vi "HEWH GEA3.vi"(8 "error in":errorcluster, 11 "Message Queues out":T4) -> (0 "error out":errorcluster)   [LabVIEW 2023]
uses:
  Tenney/support/Message Queue/All Message Queues.ctl
  Tenney/support/Message Queue/Message Cluster.ctl
  Type Definitions/HEWH GEA3 Data.ctl
  Drivers/GEA3 Toolkit/LabVIEW GEA3 Rev2 API Toolkit LV2016/Water Heating Specific/Type Definitions/GEA3 HEWH ERD Data.ctl
  Drivers/GEA3 Toolkit/LabVIEW GEA3 Rev2 API Toolkit LV2016/Water Heating Specific/Type Definitions/GEA3 HEWH Mixing Valve.ctl
  Type Definitions/HEWH GEA3 Board ID.ctl
  Drivers/GEA3 Toolkit/LabVIEW GEA3 Rev2 API Toolkit LV2016/type defs/ERD Write Data In.ctl
  Drivers/GEA3 Toolkit/LabVIEW GEA3 Rev2 API Toolkit LV2016/type defs/Data Type.ctl
  Utility/Save File/File Setup (Public)/Type Definition/Save File HEWH Heating Control Mode.ctl
  Drivers/GEA3 Toolkit/LabVIEW GEA3 Rev2 API Toolkit LV2016/Water Heating Specific/Type Definitions/GEA3 HEWH Personality.ctl
  FVIR and LDO/support/Message Queue/Enqueue Message (Single).vi
  FVIR and LDO/support/Message Queue/Message Queue.lvlib
  Drivers/GEA3 Toolkit/LabVIEW GEA3 Rev2 API Toolkit LV2016/library/GEA2_Toolkit.lvlib
  Utility/Save File/File Setup.lvlib
  Tenney/support/Message Queue/Tenney Message Queue.lvlib
panel:
  out "Loop Count":i32
  out "GEA3 Data":T1
  out "Pink Bean Board ID":string
  in  "Debug":bool
  out "Debug":string[](array[string])
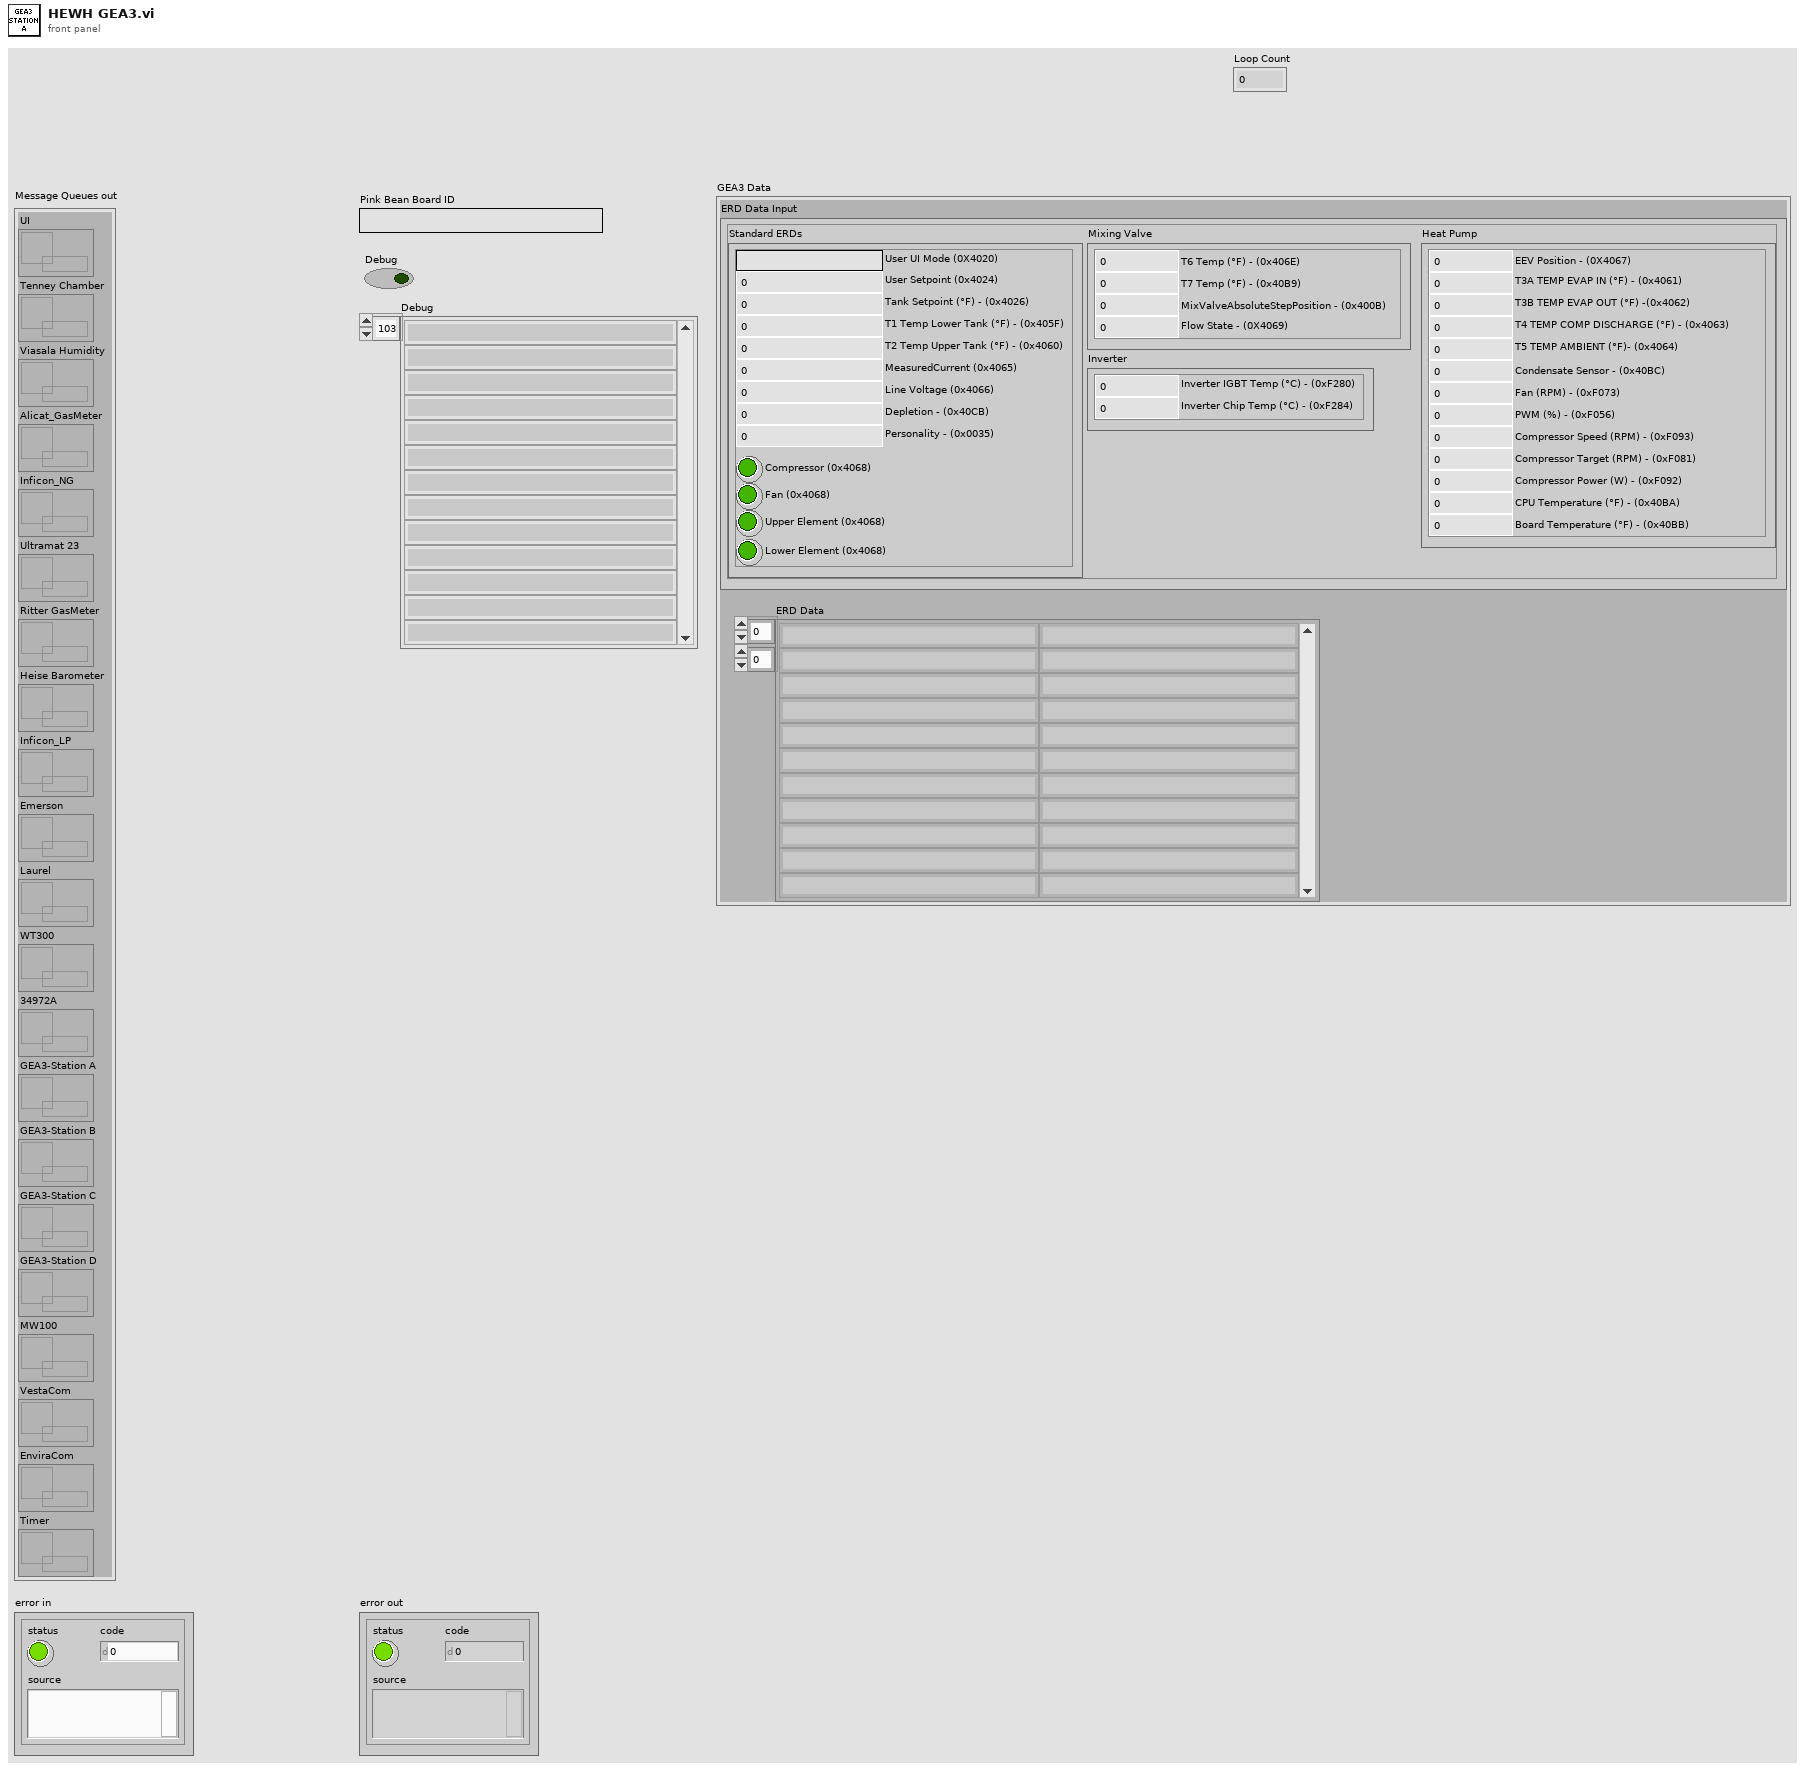
[diagram p1: front panel]
types:
  T1 = typedef "HEWH GEA3 Data.ctl" = cluster{"ERD Data Input":T2, "ERD Data":string[][]}
  T2 = typedef "GEA3 HEWH ERD Data.ctl" = cluster{"Mixing Valve":T3, "Standard ERDs":cluster{"User UI Mode (0X4020)":string, "User Setpoint (0x4024)":u16, "Compressor (0x4068)":bool, "Lower Element (0x4068)":bool, "Upper Element (0x4068)":bool, "Fan (0x4068)":bool, "T1 Temp Lower Tank (°F) - (0x405F)":dbl, "T2 Temp Upper Tank (°F) - (0x4060)":dbl, "Line Voltage (0x4066)":u16, "MeasuredCurrent (0x4065)":dbl, "Tank Setpoint (°F) - (0x4026)":u16, "Depletion - (0x40CB)":u16, "Personality - (0x0035)":u16}, "Heat Pump":cluster{"EEV Position - (0X4067)":u16, "T3A TEMP EVAP IN (°F) - (0x4061)":dbl, "T3B TEMP EVAP OUT (°F) -(0x4062)":dbl, "T4 TEMP COMP DISCHARGE (°F) - (0x4063)":dbl, "T5 TEMP AMBIENT (°F)- (0x4064)":dbl, "Condensate Sensor - (0x40BC)":u16, "Fan (RPM) - (0xF073)":u16, "PWM (%) - (0xF056)":u16, "Compressor Speed (RPM) - (0xF093)":u16, "Compressor Target (RPM) - (0xF081)":u16, "Compressor Power (W) - (0xF092)":u16, "CPU Temperature (°F) - (0x40BA)":dbl, "Board Temperature (°F) - (0x40BB)":dbl}, "Inverter":cluster{"Inverter IGBT Temp (°C) - (0xF280)":dbl, "Inverter Chip Temp (°C) - (0xF284)":dbl}}
  T3 = typedef "GEA3 HEWH Mixing Valve.ctl" = cluster{"T7 Temp (°F) - (0x40B9)":dbl, "MixValveAbsoluteStepPosition - (0x400B)":i16, "Flow State - (0X4069)":u8, "T6 Temp (°F) - (0x406E)":dbl}
  T4 = typedef "Tenney Message Queue.lvlib/All Message Queues.ctl" = cluster{"UI":refnum<queue>, "Tenney Chamber":refnum<queue>, "Viasala Humidity":refnum<queue>, "Alicat_GasMeter":refnum<queue>, "Inficon_NG":refnum<queue>, "Ultramat 23":refnum<queue>, "Ritter GasMeter":refnum<queue>, "Heise Barometer":refnum<queue>, "Inficon_LP":refnum<queue>, "Emerson":refnum<queue>, "Laurel":refnum<queue>, "WT300":refnum<queue>, "34972A":refnum<queue>, "GEA3-Station A":refnum<queue>, "GEA3-Station B":refnum<queue>, "GEA3-Station C":refnum<queue>, "GEA3-Station D":refnum<queue>, "MW100":refnum<queue>, "VestaCom":refnum<queue>, "EnviraCom":refnum<queue>, "Timer":refnum<queue>}
  T5 = typedef "HEWH GEA3 Board ID.ctl" = enum16{"Board ID - 0", "Board ID - 1", "Board ID - 2", "Board ID - 3"}
  T6 = typedef "GEA2_Toolkit.lvlib/ERD Write Data In.ctl" = cluster{"ERD Number":u16, "Data Type":T7, "Data":string}
  T7 = typedef "GEA2_Toolkit.lvlib/Data Type.ctl" = enum16{"string", "boolean", "uint8_t", "uint16_t", "uint32_t", "uint64_t", "int8_t", "int16_t", "int32_t", "int64_t"}
  T8 = typedef "File Setup.lvlib/Save File HEWH Heating Control Mode.ctl" = string
  T9 = typedef "GEA3 HEWH Personality.ctl" = string
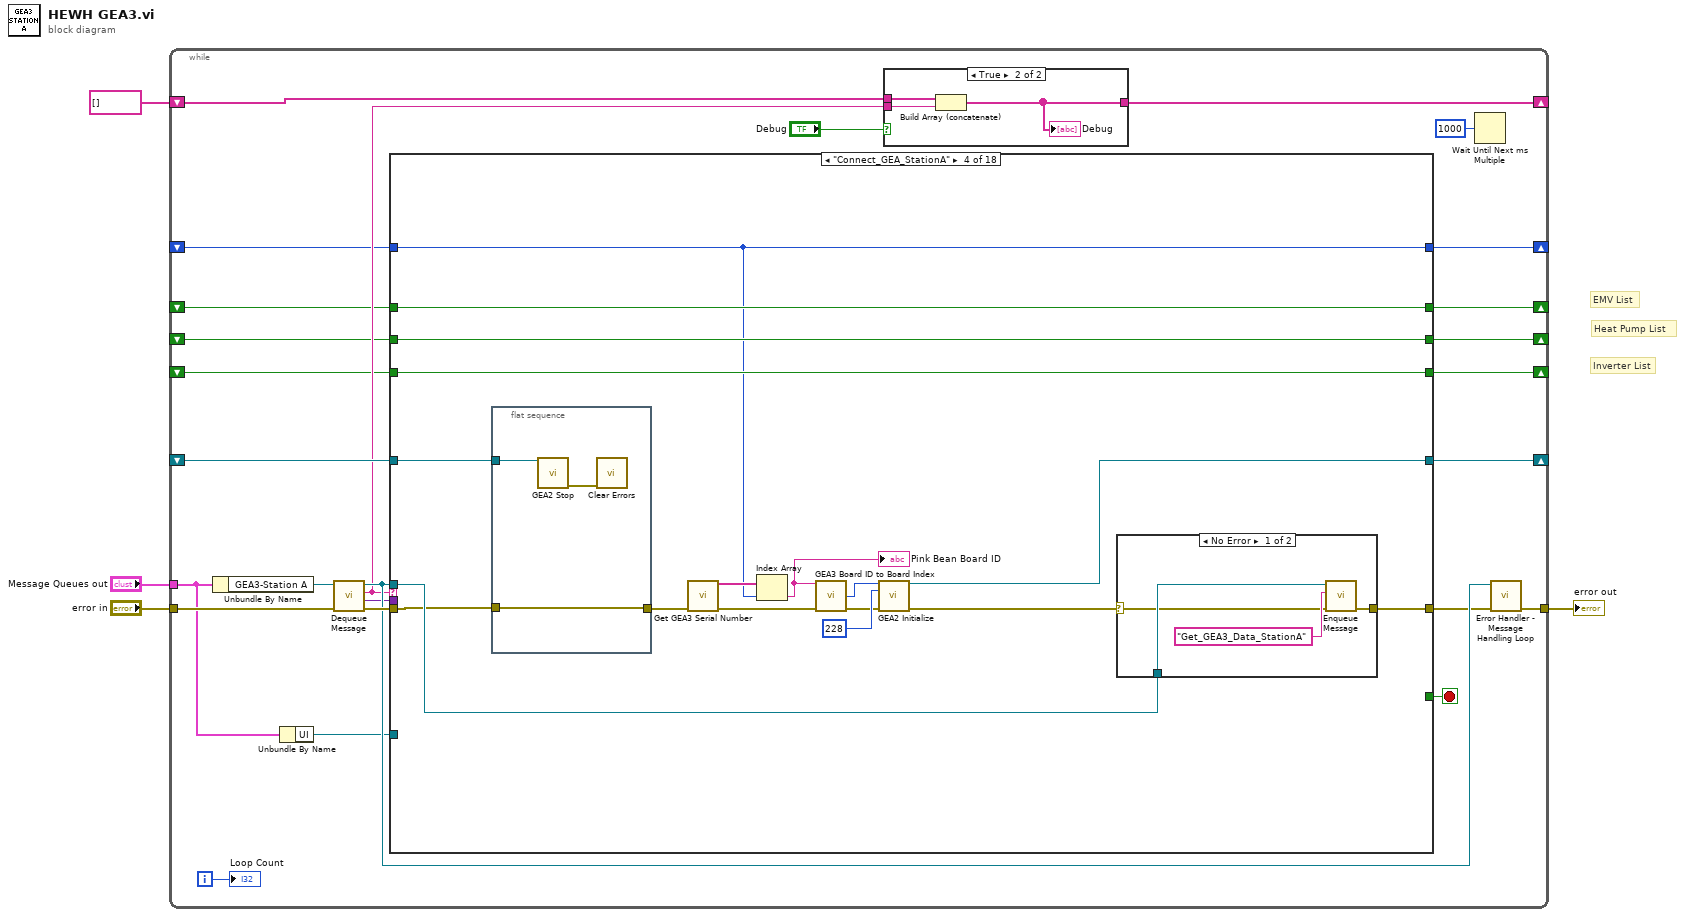
[diagram p0: block diagram]
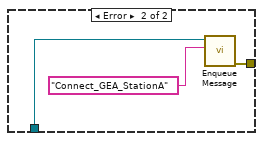
[diagram p6: hidden frame]
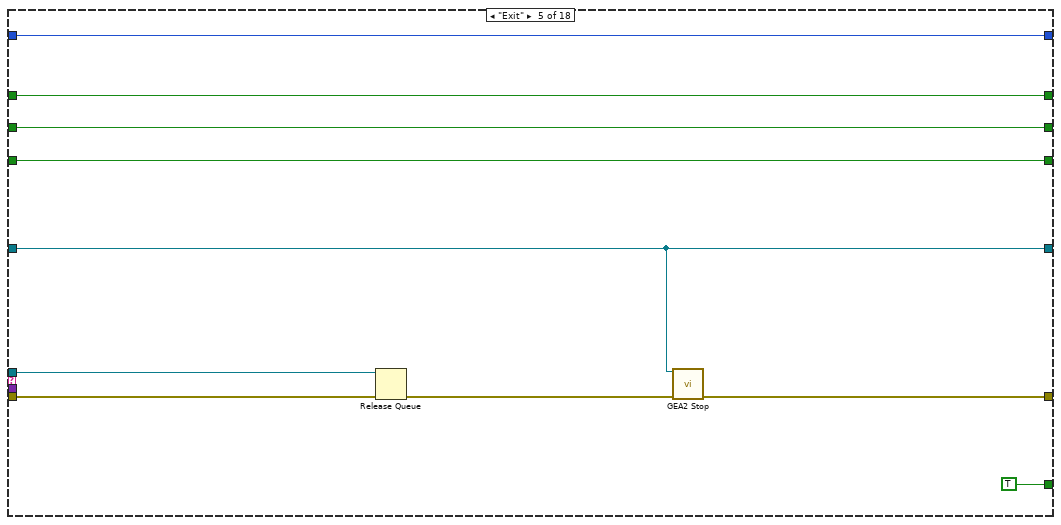
[diagram p7: hidden frame]
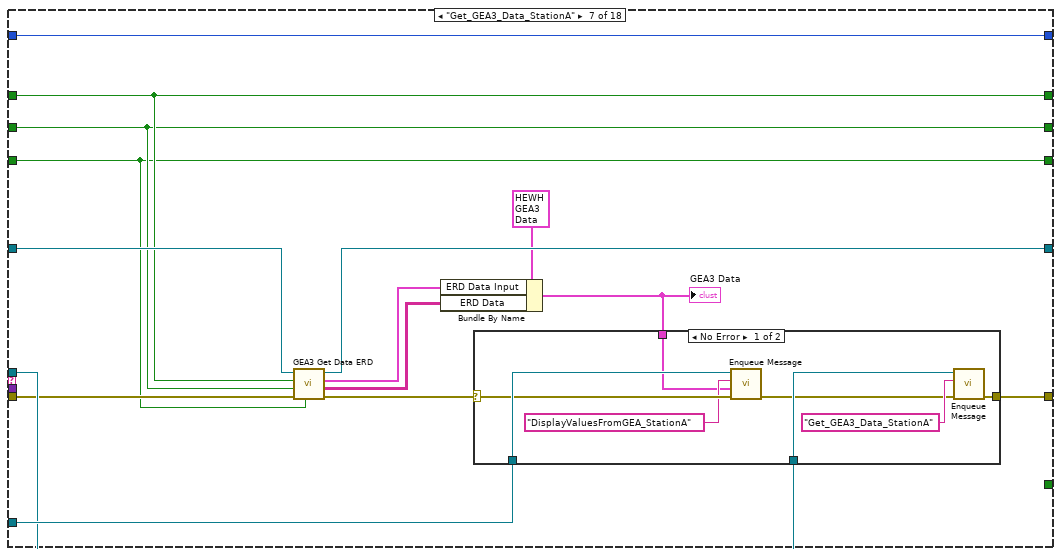
[diagram p9: hidden frame]
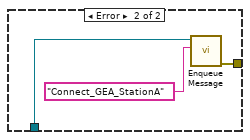
[diagram p10: hidden frame]
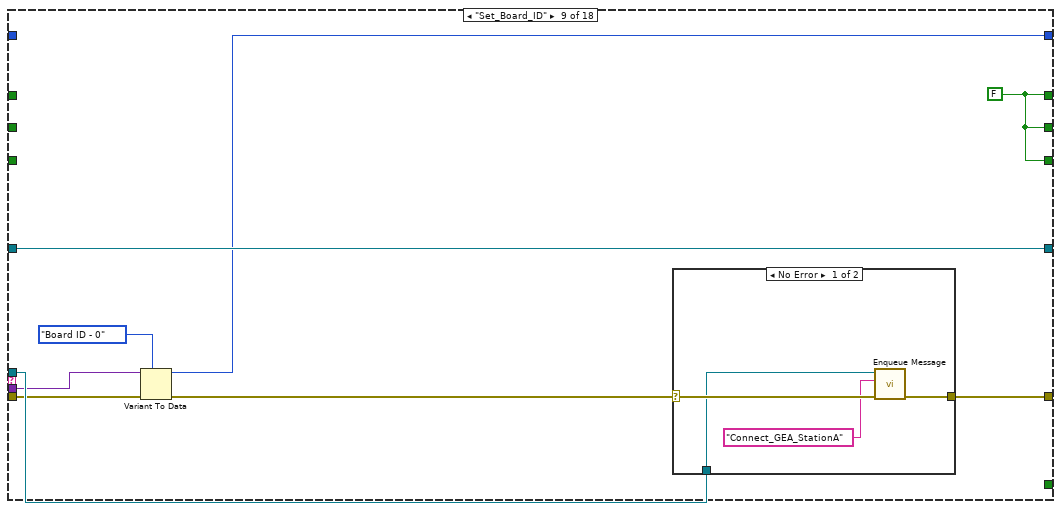
[diagram p12: hidden frame]
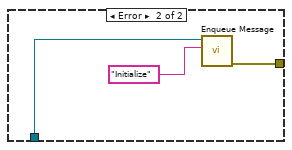
[diagram p13: hidden frame]
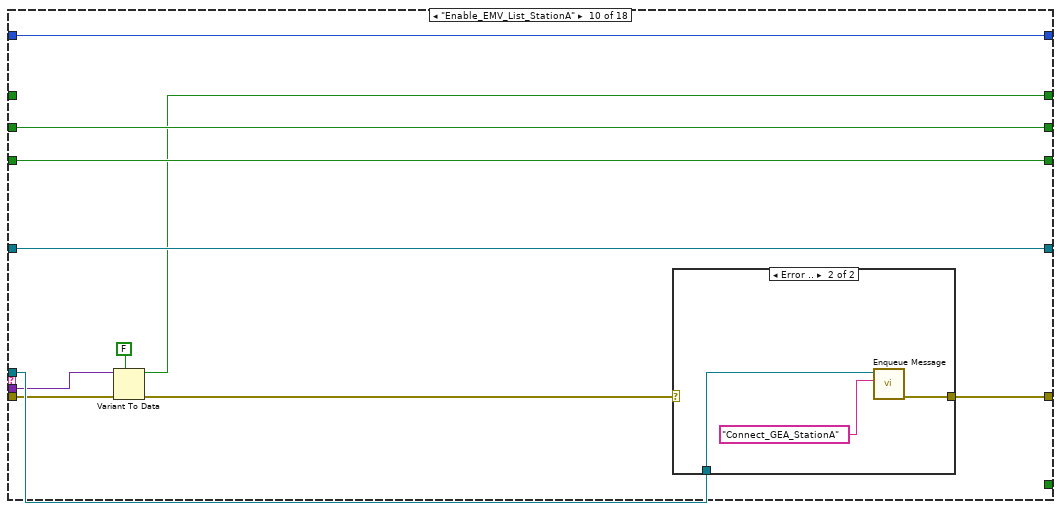
[diagram p14: hidden frame]
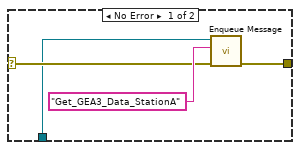
[diagram p15: hidden frame]
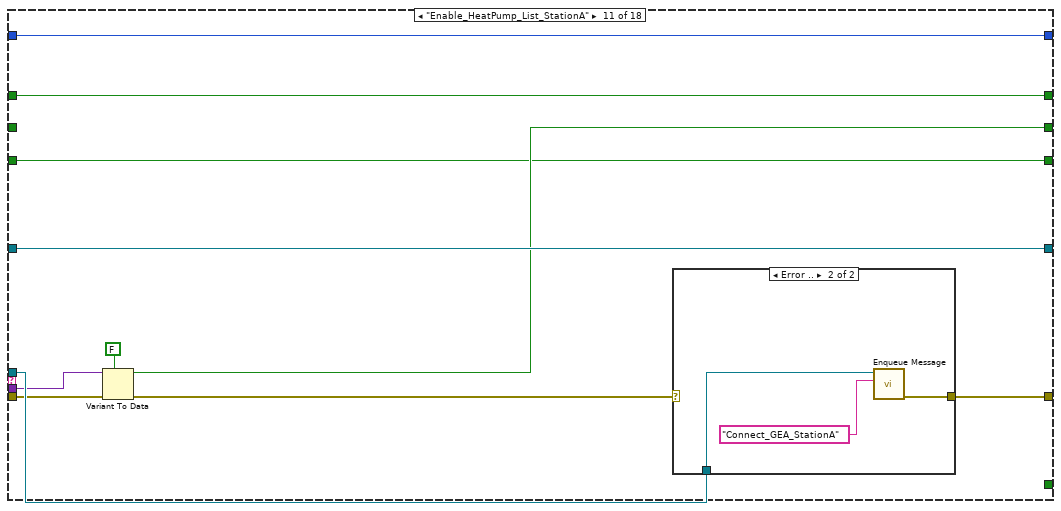
[diagram p16: hidden frame]
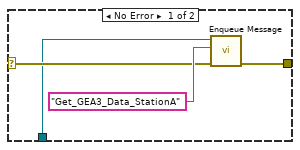
[diagram p17: hidden frame]
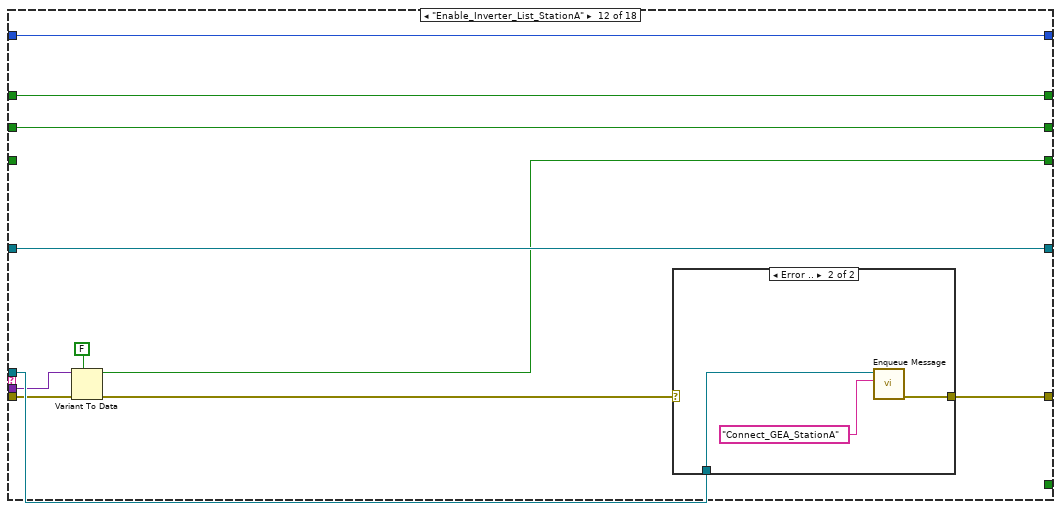
[diagram p18: hidden frame]
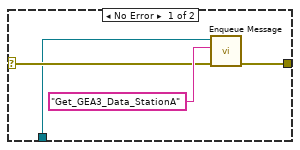
[diagram p19: hidden frame]
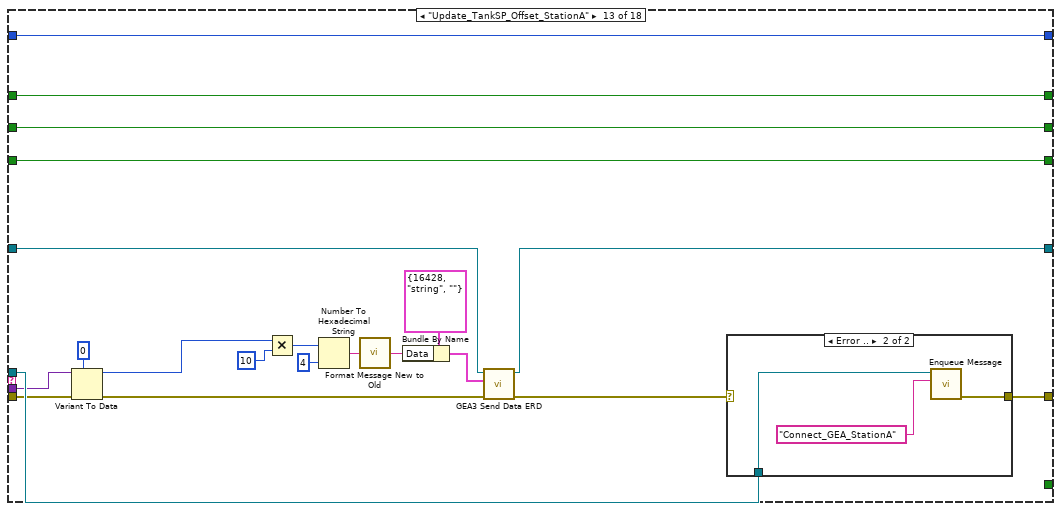
[diagram p20: hidden frame]
diagram:
  # "Inverter List"
  # "Heat Pump List"
  # "EMV List"
  n1 = while {
    tunnel: "Message Queues out" -> [w20]
    tunnel: "error in" -> [w29]
    tunnel: [w25] -> w3
    shift-right: [w23] -> _
    shift-left: _ -> [w22]
    shift-right: [w16] -> _
    shift-left: string[] [] -> [w17]
    shift-right: [w14] -> _
    shift-left: _ -> [w11]
    shift-right: [w13] -> _
    shift-left: _ -> [w10]
    shift-right: [w12] -> _
    shift-left: _ -> [w9]
    shift-right: [w7] -> _
    shift-left: _ -> [w6]
    i -> [w5]
    stop <- w27 stop-if-true
    n2 = Unbundle By Name(w20) -> ("GEA3-Station A"=w30:refnum<queue>)
    n3 = Unbundle By Name(w20) -> ("UI"=w19:refnum<queue>)
    n4 = call "Dequeue Message.vi"("error in (no error)"=w29, "Message Queue"=w30) -> ("error out"=w28:errorcluster, "Message Data"=w8:variant, "Message"=w18:string, "dup Message Queue"=w26:refnum<queue>)  [unwired: 6 in]
    n5 = case shown="\"Connect_GEA_StationA\"" w18 {
      tunnel: w28 -> [w36 w42 w51 w56 w87 w91 w107 w123 w133 w149 w168 w186 w216 w244 w272 w295 w320 w332]
      tunnel: [w36 w42 w51 w69 w82 w91 w109 w123 w136 w154 w172 w190 w218 w246 w274 w297 w322 w346] -> w24
      tunnel: [_ _ _ _ TRUE _ _ _ _ _ _ _ _ _ _ _ _ _] -> w27
      tunnel: w26 -> [_ _ _ w68 w88 _ w108 _ w135 w153 w171 w189 w217 w245 w273 w296 w321 w345]
      tunnel: [w40 w46 w52 w60 w81 w95 w105 w127 w134 w152 w170 w188 w203 w231 w265 w288 w314 w340] -> w23
      tunnel: w22 -> [w40 w46 w52 w54 w81 w95 w104 w127 w134 w152 w170 w188 w204 w232 w266 w289 w315 w341]
      tunnel: w19 -> [_ _ _ _ _ _ w110 _ _ _ _ _ _ _ _ _ _ _]
      tunnel: [w39 w45 w50 w59 w86 w94 w103 w126 w130 w145 w164 w182 w214 w242 w270 w293 w318 w344] -> w14
      tunnel: [w38 w44 w49 w58 w85 w93 w102 w125 w130 w151 w165 w181 w213 w241 w269 w292 w317 w343] -> w13
      tunnel: [w37 w43 w48 w57 w84 w92 w101 w124 w130 w150 w163 w183 w199 w227 w262 w285 w311 w338] -> w12
      tunnel: w11 -> [w39 w45 w50 w59 w86 w94 w103 w126 _ _ w164 w182 w214 w242 w270 w293 w318 w344]
      tunnel: w10 -> [w38 w44 w49 w58 w85 w93 w102 w125 _ w151 _ w181 w213 w241 w269 w292 w317 w343]
      tunnel: w9 -> [w37 w43 w48 w57 w84 w92 w101 w124 _ w150 w163 _ w199 w227 w262 w285 w311 w338]
      tunnel: w8 -> [_ _ _ _ _ _ _ _ w131 w147 w166 w184 w215 w243 w271 w294 w319 _]
      tunnel: [w35 w41 w47 w53 w80 w90 w96 w122 w128 w144 w162 w180 w198 w226 w254 w282 w305 w330] -> w7
      tunnel: w6 -> [w35 w41 w47 w53 w80 w90 w96 w122 _ w144 w162 w180 w198 w226 w254 w282 w305 w330]
      frame "---------- Setup ----------" {
      }
      frame Default {
      }
      frame "Initialize" {
      }
      frame "Connect_GEA_StationA" {
        n6 = flat-sequence {
          tunnel: w56 -> [w72]
          tunnel: [w72] -> w55
          tunnel: w54 -> [w71]
          frame #0 {
            n7 = call "GEA2 Stop.vi"("GEA2 Reference In"=w71) -> ("Error Out"=w70:errorcluster)  [unwired: 14 in]
            n8 = call <vilib>:"Clear Errors.vi"("error in (no error)"=w70) -> ()  [unwired: 5 in, 2 out]
          }
        }
        n9 = call "Get GEA3 Serial Number.vi"("Error In"=w55) -> ("GEA3 Serial Numbers"=w65:string[], "Error Out"=w64:errorcluster)  [unwired: 13 in]
        n10 = Index Array(array=w65, index=w53) -> (element=w66:string)
        "Pink Bean Board ID" <- w66
        n11 = call "GEA3 Board ID to Board Index.vi"("GEA3 Serial Number"=w66, "Error In"=w64) -> ("Board Index"=w63:i32, "Error Out"=w62:errorcluster)  [unwired: 9 in, 3 out]
        n12 = call "GEA2 Initialize.vi"("Board Index"=w63, "Source Address"=u8 228, "error in"=w62) -> ("GEA2 Reference Out"=w60:refnum<k24>, "error out"=w61:errorcluster)  [unwired: 10 in, 1 out]
        n13 = case shown="No Error" w61 {
          selector: w61 -> [w73 _]
          tunnel: [w75 w78] -> w69
          tunnel: w68 -> [w74 w77]
          frame No Error {
            n14 = call-poly "Enqueue Message.vi"("error in (no error)"=w73, "Message"="Get_GEA3_Data_StationA", "Message Queue"=w74) -> ("error out"=w75:errorcluster)  [unwired: 7 in, 1 out]
          }
          frame Error {
            n15 = call-poly "Enqueue Message.vi"("Message"="Connect_GEA_StationA", "Message Queue"=w77) -> ("error out"=w78:errorcluster)  [unwired: 8 in, 1 out]
          }
        }
      }
      frame "Exit" {
        n16 = Release Queue(queue=w88, error in (no error)=w87) -> (error out=w83:errorcluster)  [unwired: 1 in, 2 out]
        n17 = call "GEA2 Stop.vi"("GEA2 Reference In"=w81, "Error In"=w83) -> ("Error Out"=w82:errorcluster)  [unwired: 13 in]
      }
      frame "---------- Data Collection ----------" {
      }
      frame "Get_GEA3_Data_StationA" {
        n18 = call "GEA3 Get Data ERD.vi"("Enable Inverter ERD List"=w101, "error in (no error)"=w107, "Enable Heat Pump List"=w102, "Enable EMV List"=w103, ".NET Refnum in"=w104) -> ("error out"=w106:errorcluster, "ERD Data"=w99:string[][], "ERD Data Input"=w98:T2, ".NET Refnum out"=w105:refnum<k24>)  [unwired: 3 in]
        n19 = Bundle By Name(cluster=T1 {"ERD Data Input"={"Mixing Valve"={"T7 Temp (°F) - (0x40B9)"=0.0, "MixValveAbsoluteStepPosition - (0x400B)"=0, "Flow State - (0X4069)"=0, "T6 Temp (°F) - (0x406E)"=0.0}, "Standard ERDs"={"User UI Mode (0X4020)"="", "User Setpoint (0x4024)"=0, "Compressor (0x4068)"=FALSE, "Lower Element (0x4068)"=FALSE, "Upper Element (0x4068)"=FALSE, "Fan (0x4068)"=FALSE, "T1 Temp Lower Tank (°F) - (0x405F)"=0.0, "T2 Temp Upper Tank (°F) - (0x4060)"=0.0, "Line Voltage (0x4066)"=0, "MeasuredCurrent (0x4065)"=0.0, "Tank Setpoint (°F) - (0x4026)"=0, "Depletion - (0x40CB)"=0, "Personality - (0x0035)"=0}, "Heat Pump"={"EEV Position - (0X4067)"=0, "T3A TEMP EVAP IN (°F) - (0x4061)"=0.0, "T3B TEMP EVAP OUT (°F) -(0x4062)"=0.0, "T4 TEMP COMP DISCHARGE (°F) - (0x4063)"=0.0, "T5 TEMP AMBIENT (°F)- (0x4064)"=0.0, "Condensate Sensor - (0x40BC)"=0, "Fan (RPM) - (0xF073)"=0, "PWM (%) - (0xF056)"=0, "Compressor Speed (RPM) - (0xF093)"=0, "Compressor Target (RPM) - (0xF081)"=0, "Compressor Power (W) - (0xF092)"=0, "CPU Temperature (°F) - (0x40BA)"=0.0, "Board Temperature (°F) - (0x40BB)"=0.0}, "Inverter"={"Inverter IGBT Temp (°C) - (0xF280)"=0.0, "Inverter Chip Temp (°C) - (0xF284)"=0.0}}, "ERD Data"=[]} ("GEA3 Data"), "ERD Data Input"=w98, "ERD Data"=w99) -> (w97:T1)
        "GEA3 Data" <- w97
        n20 = case shown="No Error" w106 {
          selector: w106 -> [w113 _]
          tunnel: w110 -> [w118 _]
          tunnel: [w117 w120] -> w109
          tunnel: w108 -> [w116 w119]
          tunnel: w97 -> [w111 _]
          frame No Error {
            n21 = call-poly "Enqueue Message.vi"("error in (no error)"=w113, "Message Data"=w111, "Message"="DisplayValuesFromGEA_StationA", "Message Queue"=w118) -> ("error out"=w114:errorcluster)  [unwired: 6 in, 1 out]
            n22 = call-poly "Enqueue Message.vi"("error in (no error)"=w114, "Message"="Get_GEA3_Data_StationA", "Message Queue"=w116) -> ("error out"=w117:errorcluster)  [unwired: 7 in, 1 out]
          }
          frame Error {
            n23 = call-poly "Enqueue Message.vi"("Message"="Connect_GEA_StationA", "Message Queue"=w119) -> ("error out"=w120:errorcluster)  [unwired: 8 in, 1 out]
          }
        }
      }
      frame "---------- Events ----------" {
      }
      frame "Set_Board_ID" {
        w130 = FALSE
        n24 = Variant To Data(error in=w133, type=HEWH_GEA3_Board_ID."Board ID - 0" ("GEA3 Pink Bean Board Index (Station A)"), Variant=w131) -> (data=w128:T5, error out=w132:errorcluster)
        n25 = case shown="No Error" w132 {
          selector: w132 -> [w140 _]
          tunnel: [w139 w142] -> w136
          tunnel: w135 -> [w138 w141]
          frame No Error {
            n26 = call-poly "Enqueue Message.vi"("error in (no error)"=w140, "Message"="Connect_GEA_StationA", "Message Queue"=w138) -> ("error out"=w139:errorcluster)  [unwired: 7 in, 1 out]
          }
          frame Error {
            n27 = call-poly "Enqueue Message.vi"("Message"="Initialize", "Message Queue"=w141) -> ("error out"=w142:errorcluster)  [unwired: 8 in, 1 out]
          }
        }
      }
      frame "Enable_EMV_List_StationA" {
        n28 = Variant To Data(error in=w149, type=FALSE, Variant=w147) -> (data=w145:bool, error out=w148:errorcluster)
        n29 = case shown="Error .." w148 {
          selector: w148 -> [w157 _]
          tunnel: [w156 w160] -> w154
          tunnel: w153 -> [w155 w159]
          frame No Error {
            n30 = call-poly "Enqueue Message.vi"("error in (no error)"=w157, "Message"="Get_GEA3_Data_StationA", "Message Queue"=w155) -> ("error out"=w156:errorcluster)  [unwired: 7 in, 1 out]
          }
          frame Error {
            n31 = call-poly "Enqueue Message.vi"("Message"="Connect_GEA_StationA", "Message Queue"=w159) -> ("error out"=w160:errorcluster)  [unwired: 8 in, 1 out]
          }
        }
      }
      frame "Enable_HeatPump_List_StationA" {
        n32 = Variant To Data(error in=w168, type=FALSE, Variant=w166) -> (data=w165:bool, error out=w167:errorcluster)
        n33 = case shown="Error .." w167 {
          selector: w167 -> [w175 _]
          tunnel: [w174 w178] -> w172
          tunnel: w171 -> [w173 w177]
          frame No Error {
            n34 = call-poly "Enqueue Message.vi"("error in (no error)"=w175, "Message"="Get_GEA3_Data_StationA", "Message Queue"=w173) -> ("error out"=w174:errorcluster)  [unwired: 7 in, 1 out]
          }
          frame Error {
            n35 = call-poly "Enqueue Message.vi"("Message"="Connect_GEA_StationA", "Message Queue"=w177) -> ("error out"=w178:errorcluster)  [unwired: 8 in, 1 out]
          }
        }
      }
      frame "Enable_Inverter_List_StationA" {
        n36 = Variant To Data(error in=w186, type=FALSE, Variant=w184) -> (data=w183:bool, error out=w185:errorcluster)
        n37 = case shown="Error .." w185 {
          selector: w185 -> [w193 _]
          tunnel: [w192 w196] -> w190
          tunnel: w189 -> [w191 w195]
          frame No Error {
            n38 = call-poly "Enqueue Message.vi"("error in (no error)"=w193, "Message"="Get_GEA3_Data_StationA", "Message Queue"=w191) -> ("error out"=w192:errorcluster)  [unwired: 7 in, 1 out]
          }
          frame Error {
            n39 = call-poly "Enqueue Message.vi"("Message"="Connect_GEA_StationA", "Message Queue"=w195) -> ("error out"=w196:errorcluster)  [unwired: 8 in, 1 out]
          }
        }
      }
      frame "Update_TankSP_Offset_StationA" {
        n40 = Variant To Data(error in=w216, type=i16 0, Variant=w215) -> (data=w200:i16, error out=w202:errorcluster)
        n41 = Multiply(x=w200, y=i16 10) -> (x*y=w211:i16)
        n42 = Number To Hexadecimal String(1:i16 4 ("width (-)"), 2:w211) -> (0:w209:string)
        n43 = call "Format Message New to Old.vi"("Raw Message In"=w209) -> ("Conv Message Out"=w206:string)  [unwired: 14 in]
        n44 = Bundle By Name(cluster=T6 {"ERD Number"=16428, "Data Type"=enum."string", "Data"=""} ("ERD Write Data In"), "Data"=w206) -> (w205:T6)
        n45 = call "GEA3 Send Data ERD.vi"("error in (no error)"=w202, "ERD Write Data In"=w205, ".NET Refnum in"=w204) -> ("error out"=w201:errorcluster, "GEA2 Reference Out"=w203:refnum<k24>)  [unwired: 5 in, 2 out]
        n46 = case shown="Error .." w201 {
          selector: w201 -> [w221 _]
          tunnel: [w220 w224] -> w218
          tunnel: w217 -> [w219 w223]
          frame No Error {
            n47 = call-poly "Enqueue Message.vi"("error in (no error)"=w221, "Message"="Get_GEA3_Data_StationA", "Message Queue"=w219) -> ("error out"=w220:errorcluster)  [unwired: 7 in, 1 out]
          }
          frame Error {
            n48 = call-poly "Enqueue Message.vi"("Message"="Connect_GEA_StationA", "Message Queue"=w223) -> ("error out"=w224:errorcluster)  [unwired: 8 in, 1 out]
          }
        }
      }
      frame "Update_User_Setpoint_StationA" {
        n49 = Variant To Data(error in=w244, type=i16 0, Variant=w243) -> (data=w228:i16, error out=w230:errorcluster)
        n50 = Multiply(x=w228, y=i16 10) -> (x*y=w239:i16)
        n51 = Number To Hexadecimal String(1:i16 4 ("width (-)"), 2:w239) -> (0:w237:string)
        n52 = call "Format Message New to Old.vi"("Raw Message In"=w237) -> ("Conv Message Out"=w234:string)  [unwired: 14 in]
        n53 = Bundle By Name(cluster=T6 {"ERD Number"=16420, "Data Type"=enum."string", "Data"=""} ("ERD Write Data In"), "Data"=w234) -> (w233:T6)
        n54 = call "GEA3 Send Data ERD.vi"("error in (no error)"=w230, "ERD Write Data In"=w233, ".NET Refnum in"=w232) -> ("error out"=w229:errorcluster, "GEA2 Reference Out"=w231:refnum<k24>)  [unwired: 5 in, 2 out]
        n55 = case shown="Error .." w229 {
          selector: w229 -> [w249 _]
          tunnel: [w248 w252] -> w246
          tunnel: w245 -> [w247 w251]
          frame No Error {
            n56 = call-poly "Enqueue Message.vi"("error in (no error)"=w249, "Message"="Get_GEA3_Data_StationA", "Message Queue"=w247) -> ("error out"=w248:errorcluster)  [unwired: 7 in, 1 out]
          }
          frame Error {
            n57 = call-poly "Enqueue Message.vi"("Message"="Connect_GEA_StationA", "Message Queue"=w251) -> ("error out"=w252:errorcluster)  [unwired: 8 in, 1 out]
          }
        }
      }
      frame "Update_Mode_StationA" {
        n58 = Variant To Data(error in=w272, type=T8 "" ("Heating Mode."), Variant=w271) -> (data=w256:T8, error out=w264:errorcluster)
        n59 = Decimal String To Number(string=w256, default (0L)=u16 0 ("default (0 I32)")) -> (number=w260:u16)  [unwired: 1 in, 1 out]
        n60 = Number To Hexadecimal String(1:i16 2 ("width (-)"), 2:w260) -> (0:w261:string)
        n61 = call "Format Message New to Old.vi"("Raw Message In"=w261) -> ("Conv Message Out"=w255:string)  [unwired: 14 in]
        n62 = Bundle By Name(cluster=T6 {"ERD Number"=16416, "Data Type"=enum."string", "Data"=""} ("ERD Write Data In"), "Data"=w255) -> (w267:T6)
        n63 = call "GEA3 Send Data ERD.vi"("error in (no error)"=w264, "ERD Write Data In"=w267, ".NET Refnum in"=w266) -> ("error out"=w263:errorcluster, "GEA2 Reference Out"=w265:refnum<k24>)  [unwired: 5 in, 2 out]
        n64 = case shown="Error .." w263 {
          selector: w263 -> [w277 _]
          tunnel: [w276 w280] -> w274
          tunnel: w273 -> [w275 w279]
          frame No Error {
            n65 = call-poly "Enqueue Message.vi"("error in (no error)"=w277, "Message"="Get_GEA3_Data_StationA", "Message Queue"=w275) -> ("error out"=w276:errorcluster)  [unwired: 7 in, 1 out]
          }
          frame Error {
            n66 = call-poly "Enqueue Message.vi"("Message"="Connect_GEA_StationA", "Message Queue"=w279) -> ("error out"=w280:errorcluster)  [unwired: 8 in, 1 out]
          }
        }
      }
      frame "Update_Capacity_StationA" {
        n67 = Variant To Data(error in=w295, type="" ("Capacity Setting"), Variant=w294) -> (data=w283:string, error out=w287:errorcluster)
        n68 = Bundle By Name(cluster=T6 {"ERD Number"=16426, "Data Type"=enum."string", "Data"=""} ("ERD Write Data In"), "Data"=w283) -> (w290:T6)
        n69 = call "GEA3 Send Data ERD.vi"("error in (no error)"=w287, "ERD Write Data In"=w290, ".NET Refnum in"=w289) -> ("error out"=w286:errorcluster, "GEA2 Reference Out"=w288:refnum<k24>)  [unwired: 5 in, 2 out]
        n70 = case shown="Error .." w286 {
          selector: w286 -> [w300 _]
          tunnel: [w299 w303] -> w297
          tunnel: w296 -> [w298 w302]
          frame No Error {
            n71 = call-poly "Enqueue Message.vi"("error in (no error)"=w300, "Message"="Get_GEA3_Data_StationA", "Message Queue"=w298) -> ("error out"=w299:errorcluster)  [unwired: 7 in, 1 out]
          }
          frame Error {
            n72 = call-poly "Enqueue Message.vi"("Message"="Connect_GEA_StationA", "Message Queue"=w302) -> ("error out"=w303:errorcluster)  [unwired: 8 in, 1 out]
          }
        }
      }
      frame "Update_Personality_StationA" {
        n73 = Variant To Data(error in=w320, type=T9 "" ("Personality"), Variant=w319) -> (data=w308:T9, error out=w313:errorcluster)
        n74 = Bundle By Name(cluster=T6 {"ERD Number"=0, "Data Type"=enum."string", "Data"=""} ("ERD Write Data In"), "ERD Number"=u16 53, "Data Type"=Data_Type."string", "Data"=w308) -> (w316:T6)
        n75 = call "GEA3 Send Data ERD.vi"("error in (no error)"=w313, "ERD Write Data In"=w316, ".NET Refnum in"=w315) -> ("error out"=w312:errorcluster, "GEA2 Reference Out"=w314:refnum<k24>)  [unwired: 5 in, 2 out]
        n76 = case shown="Error .." w312 {
          selector: w312 -> [w325 _]
          tunnel: [w324 w328] -> w322
          tunnel: w321 -> [w323 w327]
          frame No Error {
            n77 = call-poly "Enqueue Message.vi"("error in (no error)"=w325, "Message"="Get_GEA3_Data_StationA", "Message Queue"=w323) -> ("error out"=w324:errorcluster)  [unwired: 7 in, 1 out]
          }
          frame Error {
            n78 = call-poly "Enqueue Message.vi"("Message"="Connect_GEA_StationA", "Message Queue"=w327) -> ("error out"=w328:errorcluster)  [unwired: 8 in, 1 out]
          }
        }
      }
      frame "Reset_Control_Counter_StationA" {
        n79 = Number To Hexadecimal String(1:i16 4 ("width (-)"), 2:0 ("number")) -> (0:w331:string)
        n80 = Bundle By Name(cluster=T6 {"ERD Number"=0, "Data Type"=enum."string", "Data"=""} ("ERD Write Data In"), "ERD Number"=u16 16576, "Data Type"=Data_Type."string", "Data"=w331) -> (w342:T6)
        n81 = call "GEA3 Send Data ERD.vi"("error in (no error)"=w332, "ERD Write Data In"=w342, ".NET Refnum in"=w341) -> ("error out"=w339:errorcluster, "GEA2 Reference Out"=w340:refnum<k24>)  [unwired: 5 in, 2 out]
        n82 = case shown="Error .." w339 {
          selector: w339 -> [w349 _]
          tunnel: [w348 w352] -> w346
          tunnel: w345 -> [w347 w351]
          frame No Error {
            n83 = call-poly "Enqueue Message.vi"("error in (no error)"=w349, "Message"="Get_GEA3_Data_StationA", "Message Queue"=w347) -> ("error out"=w348:errorcluster)  [unwired: 7 in, 1 out]
          }
          frame Error {
            n84 = call-poly "Enqueue Message.vi"("Message"="Connect_GEA_StationA", "Message Queue"=w351) -> ("error out"=w352:errorcluster)  [unwired: 8 in, 1 out]
          }
        }
      }
    }
    n85 = case shown="True" "Debug" {
      tunnel: w18 -> [_ w34]
      tunnel: w17 -> [w31 w33]
      tunnel: [w31 w32] -> w16
      frame False {
      }
      frame True {
        n86 = Build Array (concatenate)(w33, w34) -> (w32:string[])
        "Debug" <- w32
      }
    }
    n87 = Wait Until Next ms Multiple(millisecond multiple=u32 1000) -> ()  [unwired: 1 out]
    n88 = call "Error Handler - Message Handling Loop.vi"("error in (no error)"=w24, "Message Queue"=w26) -> ("dup error in"=w25:errorcluster)  [unwired: 8 in, 1 out]
    "Loop Count" <- w5
  }
  "error out" <- w3
